vi "OOK_FrameCapture.vi"(7 "error in (no error)":errorcluster, 9 "Trigger level":dbl format="%0.2f", 10 "session handle":refnum<k15>) -> ()   [LabVIEW 2014]
uses:
  <instrlib>/niUSRP/niUSRP Fetch Rx Data (CDB).vi
  <instrlib>/niUSRP/niUSRP Fetch Rx Data (CDB Cluster).vi
  <vilib>/Analysis/NI_AALPro.lvlib
panel:
  out "error out":errorcluster
  out "Waveform Graph":dbl[](graph)
  out "x <= y?":bool
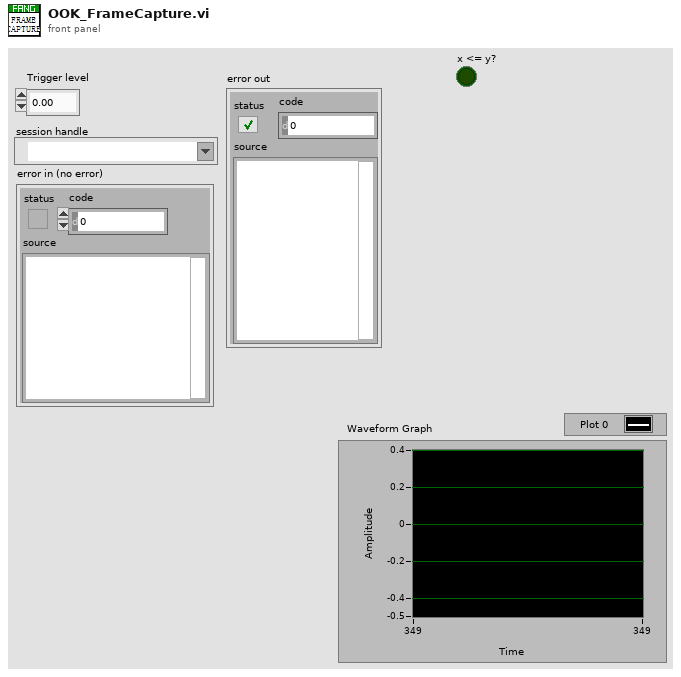
[diagram p1: front panel]
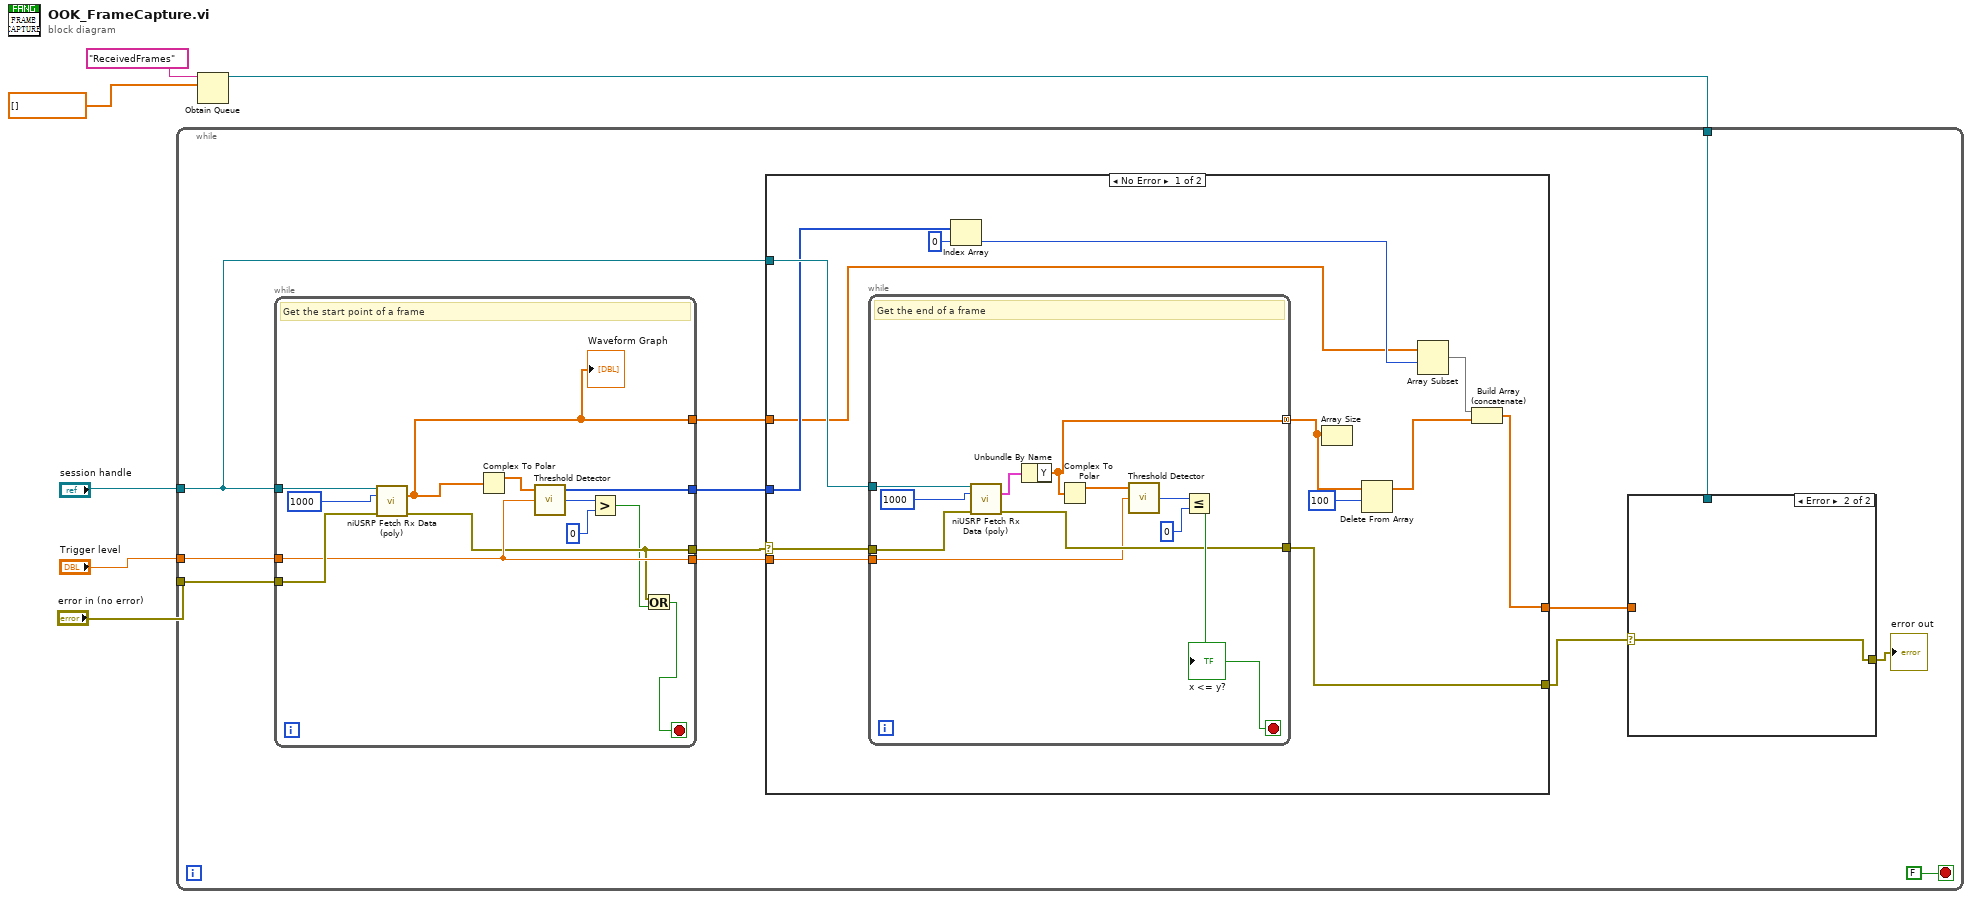
[diagram p0: block diagram]
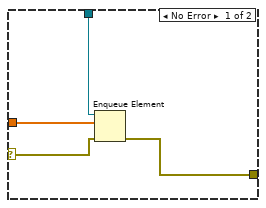
[diagram p2: hidden frame]
diagram:
  n1 = Obtain Queue(name (unnamed)="ReceivedFrames", element data type=cdb[] []) -> (queue out=w2:refnum<queue>)  [unwired: 3 in, 2 out]
  n2 = while {
    tunnel: "error in (no error)" -> [w18]
    tunnel: "Trigger level" -> [w17]
    tunnel: "session handle" -> [w16]
    tunnel: w2 -> [w11]
    stop <- FALSE stop-if-true
    n3 = while {
      tunnel: w16 -> [w58]
      tunnel: w18 -> [w61]
      tunnel: w17 -> [w56]
      tunnel: [w53] -> w12
      tunnel: [w56] -> w15
      tunnel: [w50] -> w14
      tunnel: [w54] -> w13
      stop <- w51 stop-if-true
      # "Get the start point of a frame"
      n4 = call-poly <instrlib>:"niUSRP Fetch Rx Data (poly).vi"("session handle"=w58, "number of samples"=i64 1000, "error in (no error)"=w61) -> ("data"=w50:cdb[], "error out"=w53:errorcluster)  [unwired: 9 in, 2 out]
      "Waveform Graph" <- w50
      n5 = Complex To Polar(r * e^(i*theta)=w50) -> (r=w55:dbl[])  [unwired: 1 out]
      n6 = call <vilib>:"Threshold Detector.vi"("threshold"=w56, "X"=w55) -> ("count"=w60:i32, "Indices"=w54:i32[])  [unwired: 1 in, 1 out]
      n7 = Greater?(x=w60, y=0) -> (0:w52:bool)
      n8 = Or(x=w53, y=w52) -> (x .or. y?=w51:bool)
    }
    n9 = case shown="No Error" w12 {
      selector: w12 -> [w26 w48]
      tunnel: w16 -> [w36 _]
      tunnel: [w35 w48] -> w9
      tunnel: w15 -> [w34 _]
      tunnel: w14 -> [w25 w49]
      tunnel: [w24 w49] -> w10
      tunnel: w13 -> [w30 _]
      frame No Error {
        n10 = while {
          tunnel: w36 -> [w45]
          tunnel: [w42] -> w35
          tunnel: w26 -> [w41]
          tunnel: w34 -> [w40]
          tunnel: [w37] -> w33 mode=concatenating
          stop <- w43 stop-if-true
          # "Get the end of a frame"
          n11 = call-poly <instrlib>:"niUSRP Fetch Rx Data (poly).vi"("session handle"=w45, "number of samples"=i64 1000, "error in (no error)"=w41) -> ("data"=w38:cluster{"t0":dbl, "dt":dbl, "Y":cdb[]}, "error out"=w42:errorcluster)  [unwired: 9 in, 2 out]
          n12 = Unbundle By Name(w38) -> ("Y"=w37:cdb[])
          n13 = Complex To Polar(r * e^(i*theta)=w37) -> (r=w39:dbl[])  [unwired: 1 out]
          n14 = call <vilib>:"Threshold Detector.vi"("threshold"=w40, "X"=w39) -> ("count"=w47:i32)  [unwired: 1 in, 2 out]
          n15 = Less Or Equal?(x=w47, y=0) -> (x <= y?=w43:bool)
          "x <= y?" <- w43
        }
        n16 = Index Array(array=w30, index=0) -> (element=w28:i32)
        n17 = Array Size(array=w33) -> ()  [unwired: 1 out]
        n18 = Delete From Array(array=w33, length=100) -> (array with subset deleted=w31:cdb[])  [unwired: 1 in, 1 out]
        n19 = Array Subset(array=w25, index=w28) -> (w27:cdb[])  [unwired: 1 in]
        n20 = Build Array (concatenate)(w27, w31) -> (w24:cdb[])
      }
      frame Error {
      }
    }
    n21 = case shown="Error" w9 {
      selector: w9 -> [w20 w23]
      tunnel: w11 -> [w22 _]
      tunnel: w10 -> [w21 _]
      tunnel: [w19 w23] -> w7
      frame No Error {
        n22 = Enqueue Element(queue=w22, element=w21, error in (no error)=w20) -> (error out=w19:errorcluster)  [unwired: 1 in, 2 out]
      }
      frame Error {
      }
    }
    "error out" <- w7
  }
